vi "InsertImageGreyscaleMaskARGB.vi"(6 "Greyscale Image Mask":refnum<data-value>, 7 "Offset (Default: 0,0)":T1, 8 "error in (no error)":errorcluster, 9 "ARGB Image Destination":refnum<data-value>, 10 "ARGB Image Child":refnum<data-value>, 11 "ARGB Image Parent":refnum<data-value>) -> (0 "error out":errorcluster, 3 "ARGB Image Destination (duplicate)":refnum<data-value>)   [LabVIEW 2020, in "g_ar_toolkit.image.lvlib"]
uses:
  g_ar_toolkit.image.lvlib
  Image Point (Fixed).ctl
  <vilib>/Utility/error.llb/Error Cluster From Error Code.vi
  5e3288c8-ee88-4cfe-89cf-31ceca475f5a.vi
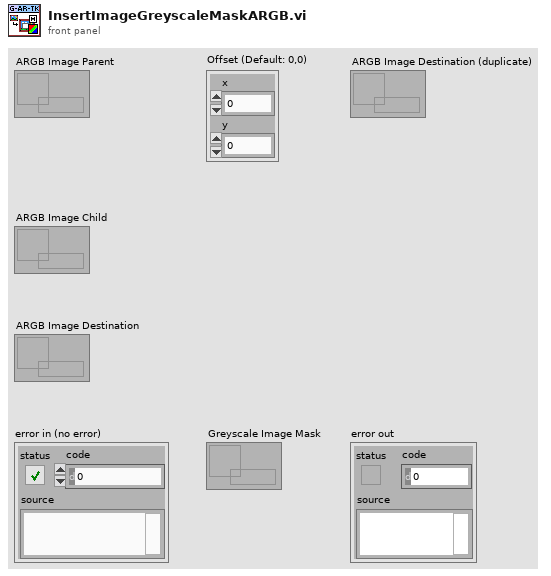
[diagram p1: front panel]
types:
  T1 = typedef "g_ar_toolkit.image.lvlib/Image Point (Fixed).ctl" = cluster{"x":i32, "y":i32}
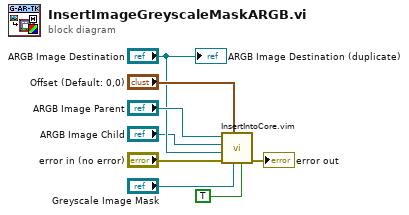
[diagram p0: block diagram]
diagram:
  n1 = call "InsertIntoCore.vim"("Has Mask"=TRUE, "Mask"="Greyscale Image Mask", "Offset"="Offset (Default: 0,0)", "error in (no error)"="error in (no error)", "Dst"="ARGB Image Destination", "Src_Child"="ARGB Image Child", "Src_Parent"="ARGB Image Parent") -> ("error out"=→"error out":errorcluster)  [unwired: 4 in]
  "ARGB Image Destination (duplicate)" <- "ARGB Image Destination"
